vi "SetTo0.vi"(10 "Longueur d'onde":dbl) -> (2 "Température 0":dbl)   [LabVIEW 2018]
uses:
  <vilib>/Analysis/NI_AALBase.lvlib
  <vilib>/Analysis/baseanly.llb/Mean (DBL).vi
  <resource>/objmgr/daqmx.rc
  <vilib>/numeric/Random Number (Range) U64.vi
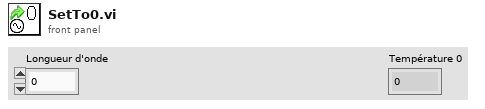
[diagram p1: front panel]
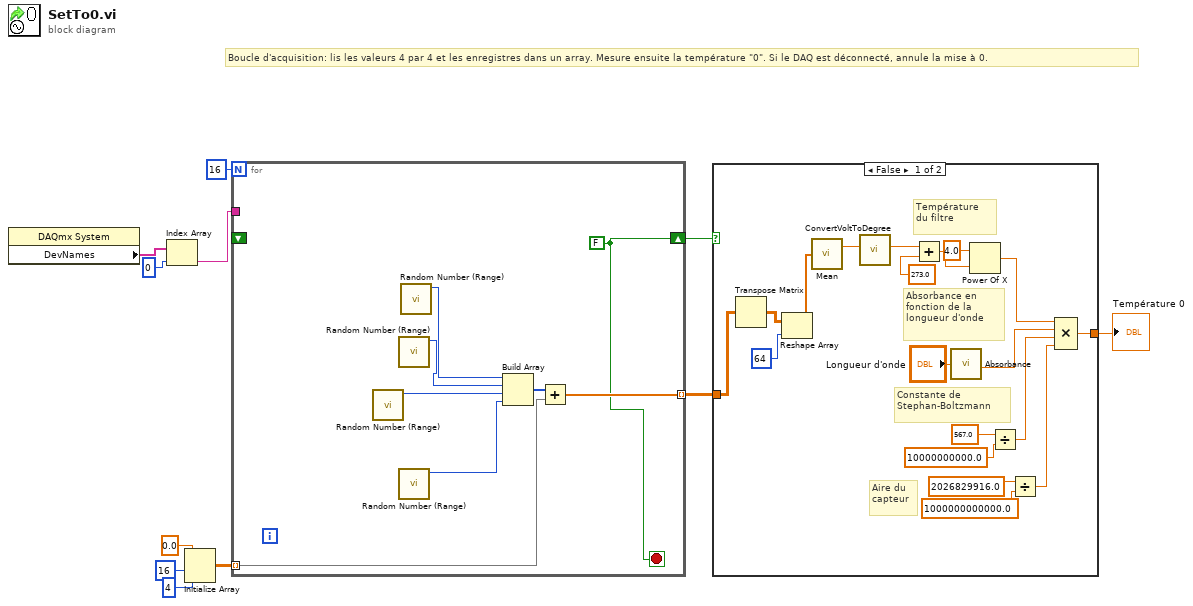
[diagram p0: block diagram]
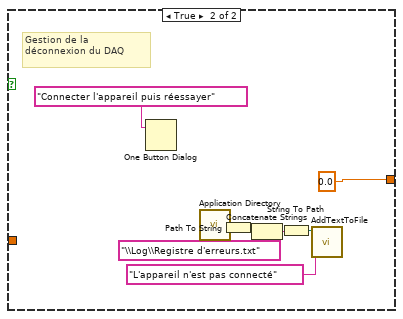
[diagram p2: hidden frame]
diagram:
  # "Boucle d'acquisition: lis les valeurs 4 par 4 et les enregistres dans un array. Mesure ensuite la température \"0\". Si le DAQ est déconnecté, annule la mise à 0."
  n1 = property class="DAQmx System"() -> ("DevNames"=w3:tag[])  [unwired: 2 in, 2 out]
  n2 = Index Array(array=w3, index=0) -> (element=w2:tag)
  n3 = Initialize Array(0.0 ("element"), 16 ("dimension size"), 4 ("dimension size")) -> (w6:dbl[][])
  n4 = for {
    N: 16 -> [_]
    shift-right: [w16] -> w10
    shift-left: _ -> [_]
    tunnel: w6 -> [w18] mode=indexing
    tunnel: [w17] -> w4 mode=indexing
    tunnel: w2 -> [_]
    stop <- w16 stop-if-true
    w16 = FALSE
    n5 = call-poly <vilib>:"Random Number (Range).vi"() -> ("number"=w13:u64)  [unwired: 11 in]
    n6 = call-poly <vilib>:"Random Number (Range).vi"() -> ("number"=w14:u64)  [unwired: 11 in]
    n7 = call-poly <vilib>:"Random Number (Range).vi"() -> ("number"=w12:u64)  [unwired: 11 in]
    n8 = call-poly <vilib>:"Random Number (Range).vi"() -> ("number"=w15:u64)  [unwired: 11 in]
    n9 = Build Array(w15, w14, w13, w12) -> (w19:u64[])
    n10 = Add(x=w19, y=w18) -> (x+y=w17:dbl[])
  }
  n11 = case shown="False" w10 {
    tunnel: w4 -> [w24 _]
    tunnel: [w20 0.0] -> w5
    frame False {
      # "Constante de \nStephan-Boltzmann"
      # "Absorbance en\nfonction de la \nlongueur d'onde"
      # "Température \ndu filtre"
      # "Aire du\ncapteur"
      n12 = Transpose Matrix(1:w24) -> (0:w25:dbl[][])
      n13 = Reshape Array(w25, 64 ("dimension size")) -> (w22:dbl[])
      n14 = call-poly <vilib>:"Mean.vi"("X"=w22) -> ("mean"=w21:dbl)  [unwired: 1 out]
      n15 = call "ConvertVoltToDegree.vi"("Tension"=w21) -> ("Température"=w30:dbl)  [unwired: 10 in]
      n16 = Add(x=w30, y=273.0) -> (x+y=w37:dbl)
      n17 = call "Absorbance.vi"("Longueur d'onde"="Longueur d'onde") -> ("absorbance"=w27:dbl)  [unwired: 10 in]
      n18 = Power Of X(1:w37, 2:4.0 ("y")) -> (0:w26:dbl)
      n19 = Divide(x=567.0, y=10000000000.0) -> (x/y=w28:dbl)
      n20 = Divide(x=2026829916.0, y=1000000000000.0) -> (x/y=w29:dbl)
      n21 = Compound Arithmetic op=MULTIPLY(w26, w27, w28, w29) -> (w20:dbl)
    }
    frame True {
      # "Gestion de la \ndéconnexion du DAQ"
      n22 = One Button Dialog(message="Connecter l'appareil puis réessayer") -> ()  [unwired: 1 in, 1 out]
      n23 = call <vilib>:"Application Directory.vi"() -> ("Application Directory"=w42:path)
      n24 = Path To String(path=w42) -> (string=w43:string)
      n25 = Concatenate Strings(w43, "\\Log\\Registre d'erreurs.txt") -> (w44:string)
      n26 = String To Path(string=w44) -> (path=w40:path)
      n27 = call "AddTextToFile.vi"("Ajouter du texte"="L'appareil n'est pas connecté", "Fichier"=w40) -> ()  [unwired: 10 in]
    }
  }
  "Température 0" <- w5
